vi "Core-InitializeUserEvents.vi"(6 "Cmd(Initialize)":enum16{"Initialize", "UnInitialize"}(ring), 8 "ErrI(No Error)":errorcluster) -> (0 "ErrO":errorcluster, 3 "User Events":T1, 5 "User Events\nRefnum":refnum<event-registration>)   [LabVIEW 2020]
doc: "Initialize or Uninitialize the user events.\n- if \"Cmd\" was set to \"Initialize\", the user event GUI::Initialize and GUI::User1 will be created and registered;\n- if \"Cmd\" was set to \"UnInitialize\", then user event GUI::Initialize and GUI::User1 will be destroyed and Unregistered;\n\nNotes:\n- SR were used to record the initialized results.\nIf vi was called by input \"UnInitialize\" after events has been initialized,\nit will close the events by the event refnum which been stored in SRs \n- You can add code here if you want to add more loop in framework."
panel:
  # "Outputs"
  # "Inputs"
  # ":: Modularized Parallism Templete ::\n- Initialize/Uninitialize User Events-\nby: Gaoke Yang <gaoke.yang@yahoo.com>\nhttp://www.mViAcademy.com\nCopyright (C) 2010, mVi Academy All Rights Reserved"
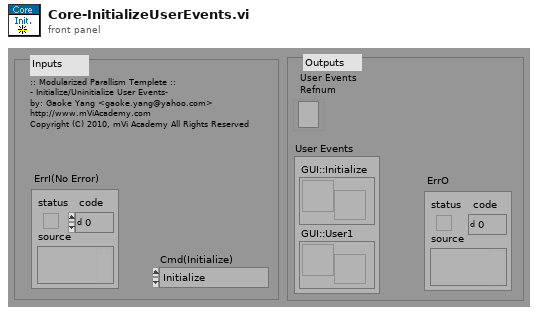
[diagram p1: front panel]
types:
  T1 = cluster{"GUI::Initialize":refnum<user-event>, "GUI::User1":refnum<user-event>}
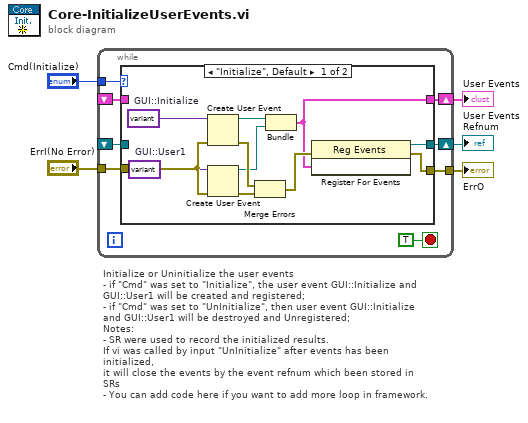
[diagram p0: block diagram]
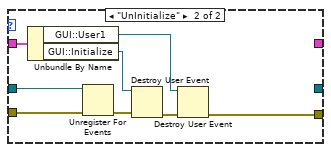
[diagram p2: hidden frame]
diagram:
  # "Initialize or Uninitialize the user events\n- if \"Cmd\" was set to \"Initialize\", the user event GUI::Initialize and GUI::User1 will be created and registered;\n- if \"Cmd\" was set to \"UnInitialize\", then user event GUI::Initialize and GUI::User1 will be destroyed and Unregistered;\nNotes:\n- SR were used to record the initialized results.\nIf vi was called by input \"UnInitialize\" after events has been initialized,\nit will close the events by the event refnum which been stored in SRs \n- You can add code here if you want to add more loop in framework."
  n1 = while {
    tunnel: "Cmd(Initialize)" -> [w11]
    tunnel: [w9] -> w4
    tunnel: "ErrI(No Error)" -> [w8]
    shift-right: [w13] -> w1
    shift-left: _ -> [w7]
    shift-right: [w10] -> w2
    shift-left: _ -> [w6]
    stop <- TRUE stop-if-true
    n2 = case shown="\"Initialize\", Default" w11 {
      tunnel: [w20 _] -> w13
      tunnel: [w19 _] -> w10
      tunnel: [w14 w25] -> w9
      tunnel: w8 -> [w18 w30]
      tunnel: w7 -> [_ w32]
      tunnel: w6 -> [_ w31]
      frame "Initialize", Default {
        w15 = variant  # GUI::User1
        w21 = variant  # GUI::Initialize
        n3 = Create User Event(user event datatype=w21, error in=w18) -> (user event=w23:refnum<user-event>, error out=w24:errorcluster)
        n4 = Create User Event(user event datatype=w15, error in=w18) -> (user event=w16:refnum<user-event>, error out=w17:errorcluster)
        n5 = Merge Errors(w24, w17) -> (w22:errorcluster)
        n6 = Bundle("GUI::Initialize"=w23, "GUI::User1"=w16) -> (w19:T1)  [unwired: 1 in]
        n7 = register-events(error in=w22, w19) -> (reference out=w20:refnum<event-registration>, error out=w14:errorcluster)  [unwired: 1 in]
      }
      frame "UnInitialize" {
        n8 = Unbundle By Name(w31) -> ("GUI::User1"=w26:refnum<user-event>, "GUI::Initialize"=w28:refnum<user-event>)
        n9 = Unregister For Events(event registration refnum=w32, error in=w30) -> (error out=w29:errorcluster)
        n10 = Destroy User Event(user event=w28, error in=w29) -> (error out=w27:errorcluster)
        n11 = Destroy User Event(user event=w26, error in=w27) -> (error out=w25:errorcluster)
      }
    }
  }
  "ErrO" <- w4
  "User Events" <- w2
  "User Events\nRefnum" <- w1
